vi "Centrowanie położenia.vi"(10 "Ostatnie położenie robota":cluster{"Pixel x":i16, "Pixel y":i16}, 11 "Mapa z wprowadzonym punktem":refnum<vi>) -> (2 "Przesunięcie wycentrowane":T1)   [LabVIEW 2015, in "Biblioteka moduł map v3.lvlib" / "Obsługa grafiki mapy.lvlib"]
uses:
  <vilib>/Utility/miscctls.llb/LVPoint32TypeDef.ctl
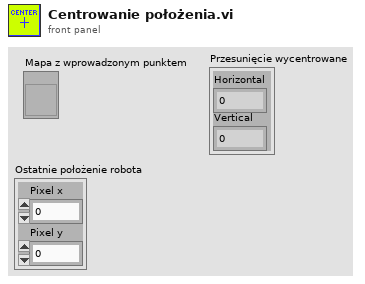
[diagram p1: front panel]
types:
  T1 = typedef "LVPoint32TypeDef.ctl" = cluster{"Horizontal":i32, "Vertical":i32}
  T2 = typedef "LVBoundsTypeDef.ctl" = cluster{"Width":u32, "Height":u32}
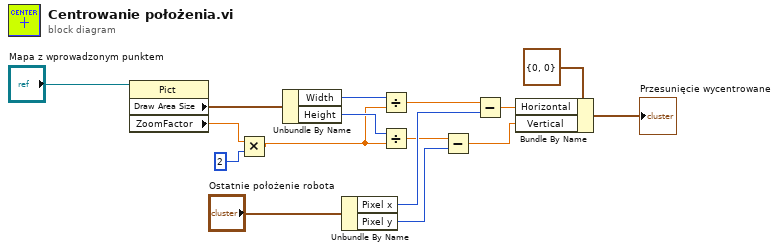
[diagram p0: block diagram]
diagram:
  n1 = property class="Pict"(reference="Mapa z wprowadzonym punktem") -> ("Draw Area Size"=w4:T2, "ZoomFactor"=w3:sgl)  [unwired: 1 in, 2 out]
  n2 = Multiply(x=w3, y=u32 2) -> (x*y=w1:sgl)
  n3 = Unbundle By Name(w4) -> ("Width"=w6:u32, "Height"=w7:u32)
  n4 = Unbundle By Name("Ostatnie położenie robota") -> ("Pixel x"=w13:i16, "Pixel y"=w14:i16)
  n5 = Divide(x=w6, y=w1) -> (x/y=w8:sgl)
  n6 = Divide(x=w7, y=w1) -> (x/y=w9:sgl)
  n7 = Subtract(x=w9, y=w14) -> (x-y=w11:sgl)
  n8 = Subtract(x=w8, y=w13) -> (x-y=w10:sgl)
  n9 = Bundle By Name(cluster=T1 {"Horizontal"=0, "Vertical"=0} ("input cluster"), "Horizontal"=w10, "Vertical"=w11) -> (→"Przesunięcie wycentrowane":T1)
